vi "get channel info.vi"(8 "error in (no error)":errorcluster, 11 "Item Ref in":T1 format="%.0x") -> (0 "error out":errorcluster, 1 "Outputs":T2, 2 "Inputs":T2, 3 "Item Ref out":T1 format="%.0x")   [LabVIEW 2015, in "Modbus Master System Explorer.lvlib"]
uses:
  Modbus Master System Explorer.lvlib
  Shared/Controls/Data Model/Channel Data.ctl
  Shared/Controls/Data Model/Channel.ctl
  Modbus Type.ctl
  <vilib>/NI Veristand/Custom Device API/Custom Device Channel Type.ctl
  Shared/Controls/Data Model/Mapping.ctl
  Shared/Controls/Data Model/DataType.ctl
  <vilib>/NI Veristand/Custom Device API/Custom Device Item Ref.ctl
  <vilib>/NI VeriStand/Custom Device API/Custom Device API.lvlib
  Shared/Modbus Master Shared.lvlib
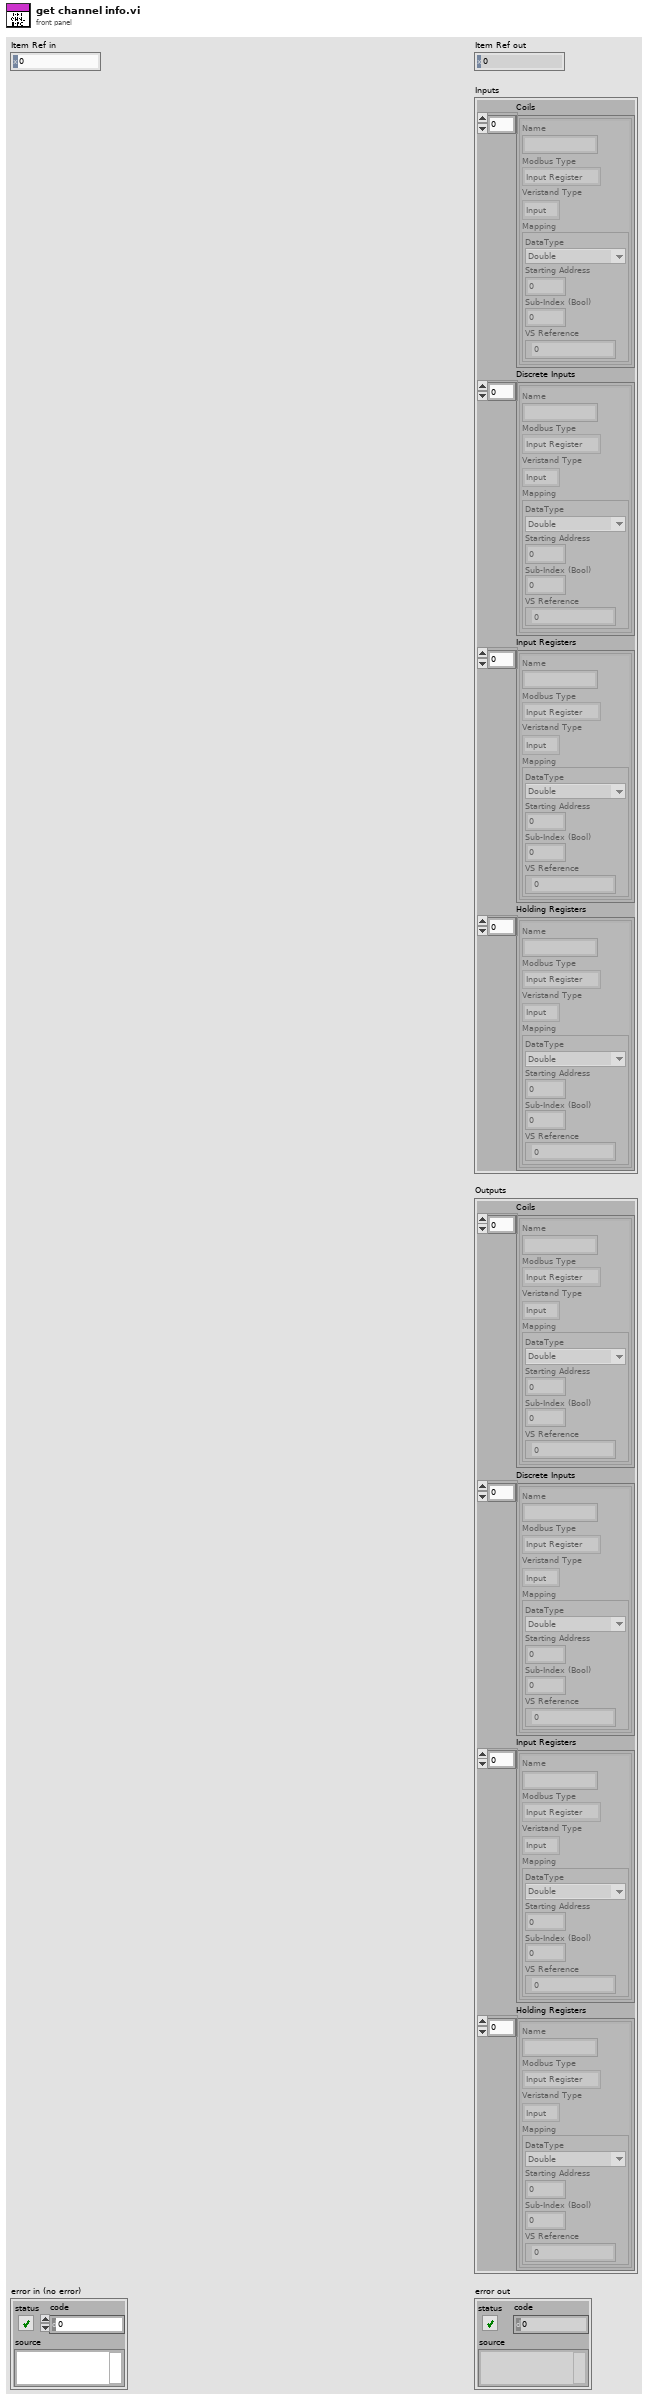
[diagram p1: front panel]
types:
  T1 = typedef "Custom Device API.lvlib/Custom Device Item Ref.ctl" = u64
  T2 = typedef "Modbus Master Shared.lvlib/Channel Data.ctl" = cluster{"Coils":T3[], "Discrete Inputs":T3[], "Input Registers":T3[], "Holding Registers":T3[]}
  T3 = typedef "Modbus Master Shared.lvlib/Channel.ctl" = cluster{"Name":string, "Modbus Type":T4, "Veristand Type":T5, "Mapping":T6}
  T4 = typedef "Modbus Master Shared.lvlib/Modbus Type.ctl" = enum16{"Coil", "Discrete Input", "Holding Register", "Input Register"}
  T5 = typedef "Custom Device API.lvlib/Custom Device Channel Type.ctl" = enum16{"Input", "Output"}
  T6 = typedef "Modbus Master Shared.lvlib/Mapping.ctl" = cluster{"DataType":T7, "Starting Address":u16, "Sub-Index (Bool)":u16, "VS Reference":T1}
  T7 = typedef "Modbus Master Shared.lvlib/DataType.ctl" = enum16{"Double", "Single", "I64", "I32", "I16", "I8", "U64", "U32", "U16", "U8", "Boolean"}
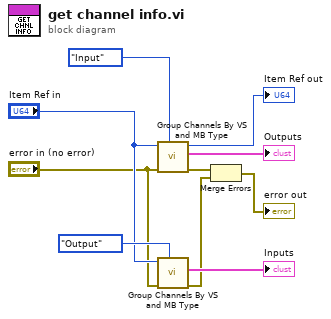
[diagram p0: block diagram]
diagram:
  n1 = call "Group Channels By VS and MB Type.vi"("Channel Type"=Custom_Device_Channel_Type."Input", "error in (no error)"="error in (no error)", "Item Ref in"="Item Ref in") -> ("error out"=w9:errorcluster, "Channels"=→"Outputs":T2, "Device Ref out"=→"Item Ref out":T1)  [unwired: 6 in]
  n2 = call "Group Channels By VS and MB Type.vi"("Channel Type"=Custom_Device_Channel_Type."Output", "error in (no error)"="error in (no error)", "Item Ref in"="Item Ref in") -> ("error out"=w1:errorcluster, "Channels"=→"Inputs":T2)  [unwired: 6 in, 1 out]
  n3 = Merge Errors(w9, w1) -> (→"error out":errorcluster)
